vi "ni579x Initialize.vi"(0 "Register Bus":T1, 7 "re-initialize?":bool, 11 "Error In":errorcluster) -> (4 "Register Bus (out)":T1, 15 "Error Out":errorcluster)   [LabVIEW 2015, in "ni579x Config v2 Host.lvlib"]
uses:
  <instrlib>/ni579x/Config/v2/Host/ni579x Config v2 Host.lvlib
  <instrlib>/_niInstr/Register Bus/v0/Host/Public/Register Bus Session.ctl
  <instrlib>/_niInstr/Register Bus/v0/Host/Private/Session Data.ctl
  <instrlib>/ni579x/Config/v2/Shared/Types/ni579x User Command.ctl
  <instrlib>/ni579x/Config/v2/Shared/Types/ni579x User Command ID.ctl
  <instrlib>/ni579x/Config/v2/Shared/ni579x Config v2 Shared.lvlib
  <instrlib>/_niInstr/Register Bus/v0/Host/niInstr Register Bus v0 Host.lvlib
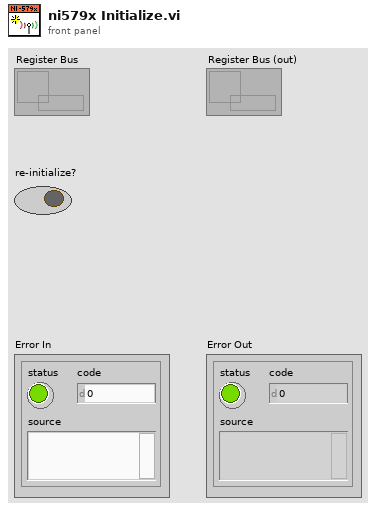
[diagram p1: front panel]
types:
  T1 = typedef "niInstr Register Bus v0 Host.lvlib/Register Bus Session.ctl" = refnum<queue>
  T2 = typedef "ni579x Config v2 Shared.lvlib/ni579x User Command.ctl" = cluster{"User Data 0":u8, "User Data 1":u8, "User Command ID":T3}
  T3 = typedef "ni579x Config v2 Shared.lvlib/ni579x User Command ID.ctl" = u8
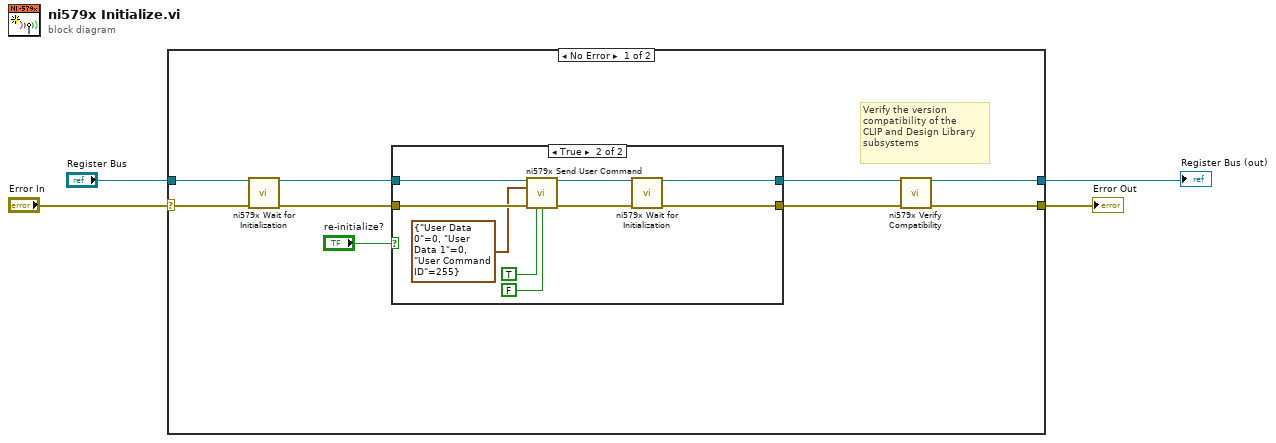
[diagram p0: block diagram]
diagram:
  n1 = case shown="No Error" "Error In" {
    selector: "Error In" -> [w11 w26]
    tunnel: [w5 w26] -> w4
    tunnel: "Register Bus" -> [w12 w25]
    tunnel: [w6 w25] -> w1
    frame No Error {
      # "Verify the version\ncompatibility of the \nCLIP and Design Library\nsubsystems"
      n2 = call <instrlib>:"ni579x Wait for Initialization.vi"("Register Bus"=w12, "Error In"=w11) -> ("Register Bus (out)"=w10:T1, "Error Out"=w9:errorcluster)  [unwired: 12 in]
      n3 = case shown="True" "re-initialize?" {
        tunnel: w10 -> [w15 w24]
        tunnel: w9 -> [w14 w23]
        tunnel: [w15 w18] -> w8
        tunnel: [w14 w17] -> w7
        frame False {
        }
        frame True {
          n4 = call <instrlib>:"ni579x Send User Command.vi"("Register Bus"=w24, "User Command"=T2 {"User Data 0"=0, "User Data 1"=0, "User Command ID"=255}, "Error In"=w23, "wait for completion?"=TRUE, "read return values?"=FALSE) -> ("Register Bus (out)"=w20:T1, "Error Out"=w19:errorcluster)  [unwired: 6 in, 3 out]
          n5 = call <instrlib>:"ni579x Wait for Initialization.vi"("Register Bus"=w20, "Error In"=w19) -> ("Register Bus (out)"=w18:T1, "Error Out"=w17:errorcluster)  [unwired: 12 in]
        }
      }
      n6 = call <instrlib>:"ni579x Verify Compatibility.vi"("Register Bus"=w8, "Error In"=w7) -> ("Register Bus (out)"=w6:T1, "Error Out"=w5:errorcluster)  [unwired: 12 in]
    }
    frame Error {
    }
  }
  "Register Bus (out)" <- w1
  "Error Out" <- w4
